vi "xcorr bkp nico SR.vi"(4 "shift":u8, 5 "Pulse Energy":fxp<+,32,0>=0.99609375, 6 "N":u8, 7 "y":u32, 8 "x":u32, 9 "enable":bool, 10 "lag":u16) -> (1 "Rxy valid":bool, 2 "Rxy":u64, 3 "trigger":bool)   [LabVIEW 2017]
uses:
  <vilib>/rvi/FXPMathLib/basic elements/FxpDiscreteDelay/XNode/nifxpmath_DiscreteDelay.xnode
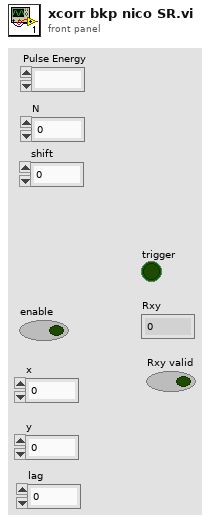
[diagram p1: front panel]
types:
  T1 = cluster{"Q[0]":bool, "Q[1]":bool, "Q[2]":bool, "Q[3]":bool, "Q[4]":bool, "Q[5]":bool, "Q[6]":bool, "Q[7]":bool, "Q[8]":bool, "Q[9]":bool, "Q[10]":bool, "Q[11]":bool, "Q[12]":bool}
  T2 = cluster{"out":u64, "Q":u64, "Q":u64, "Q":u64, "Q":u64, "Q":u64, "Q":u64, "Q":u64, "Q":u64, "Q":u64, "Q":u64, "Q":u64, "Q":u64}
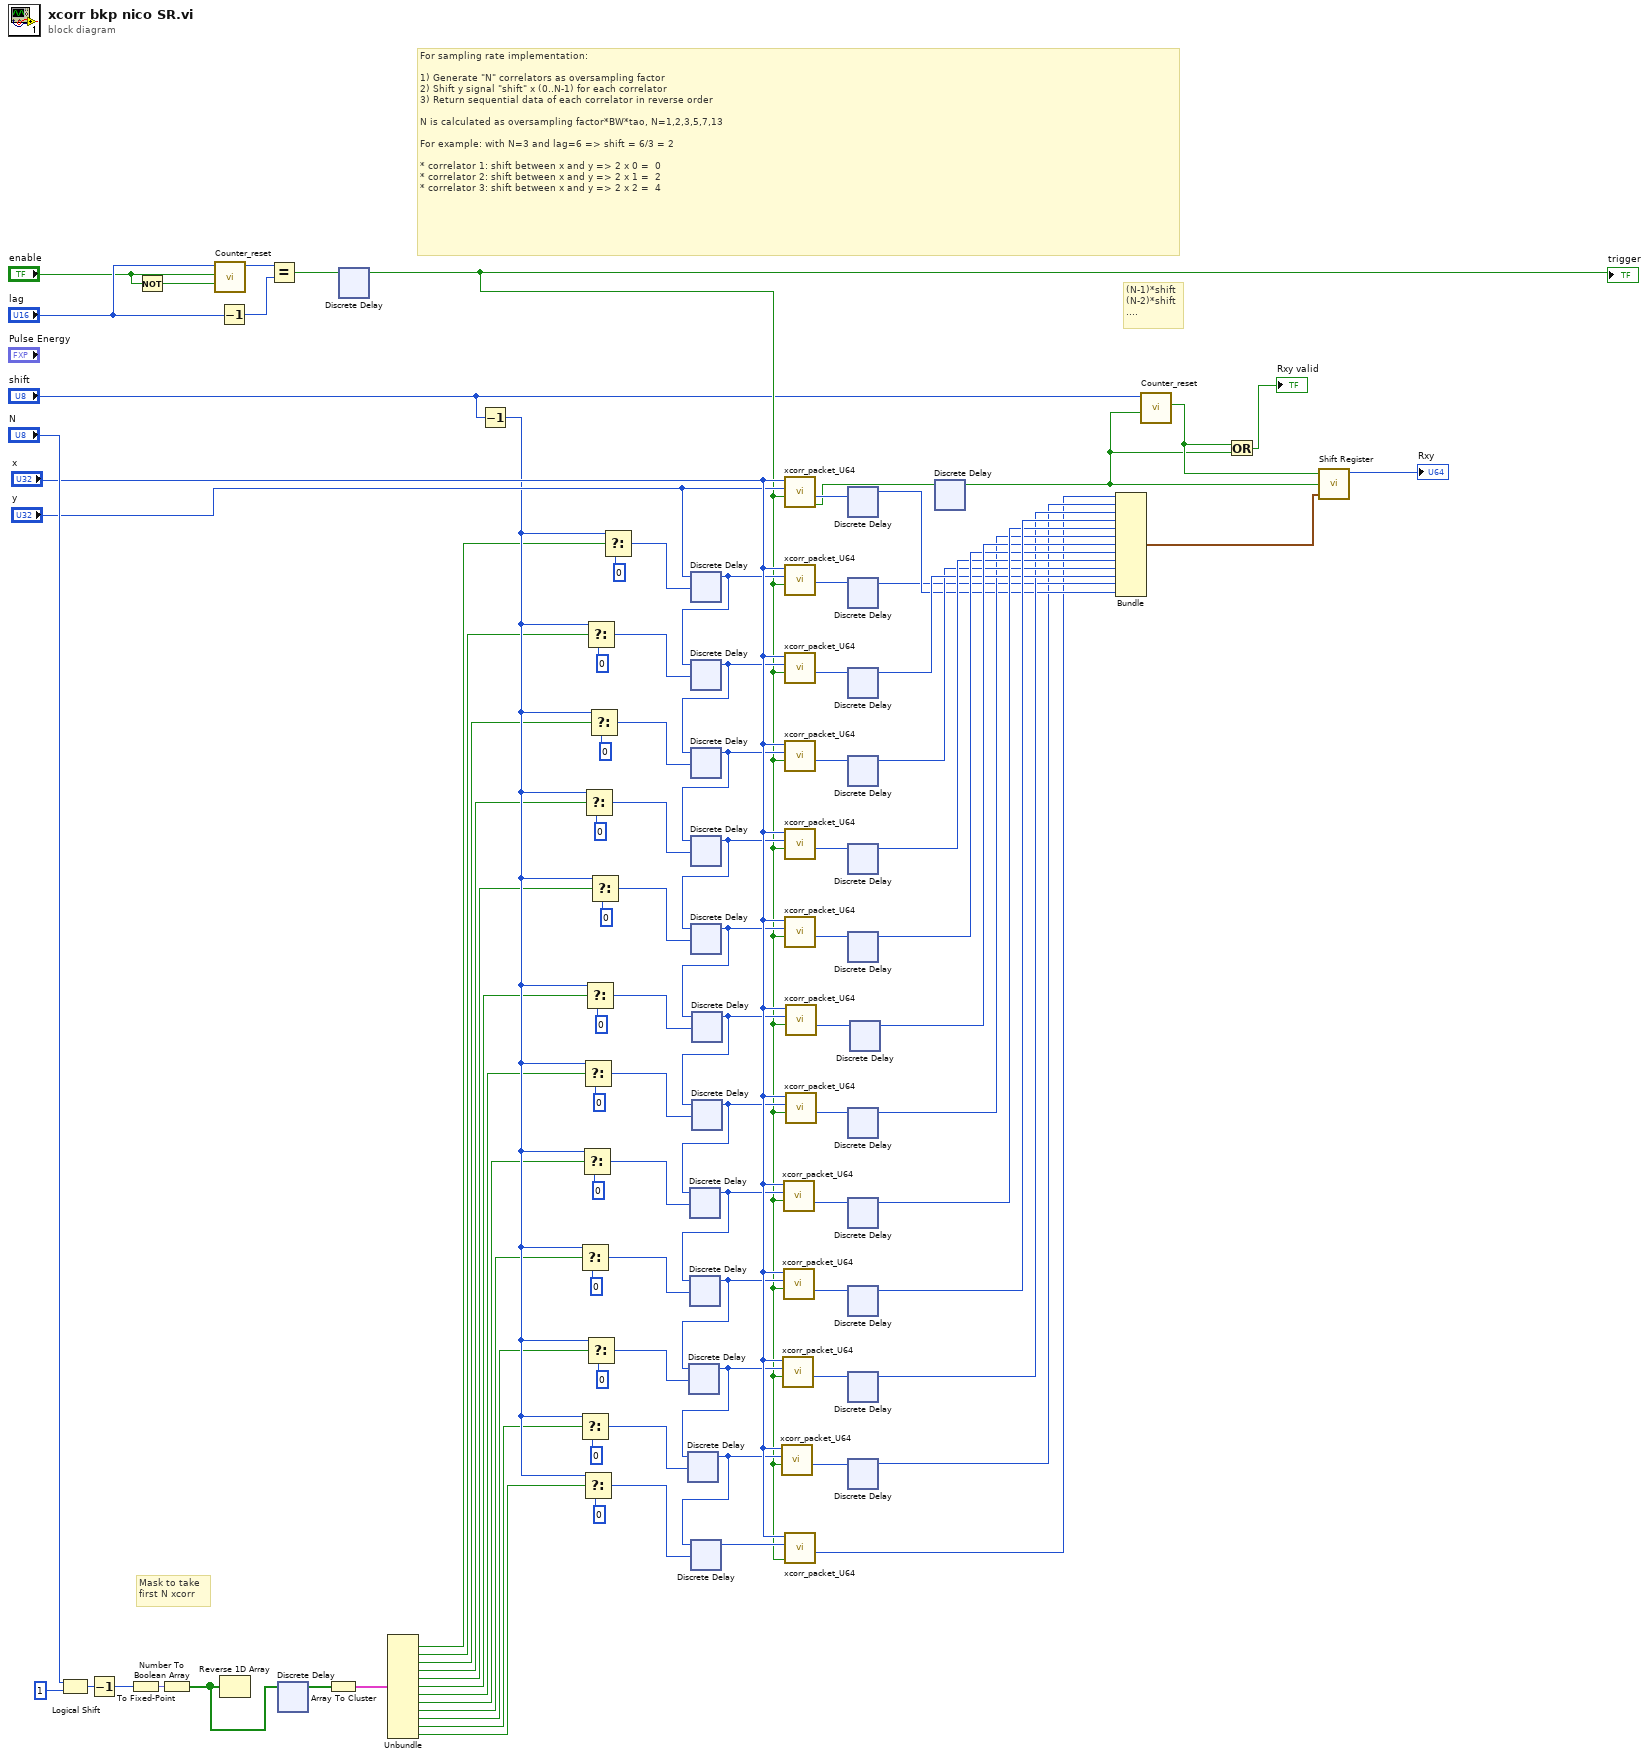
[diagram p0: block diagram]
diagram:
  # "(N-1)*shift\n(N-2)*shift\n...."
  # "Mask to take \nfirst N xcorr"
  # "For sampling rate implementation:\n\n1) Generate \"N\" correlators as oversampling factor\n2) Shift y signal \"shift\" x (0..N-1) for each correlator\n3) Return sequential data of each correlator in reverse order\n\nN is calculated as oversampling factor*BW*tao, N=1,2,3,5,7,13\n\nFor example: with N=3 and lag=6 => shift = 6/3 = 2\n\n* correlator 1: shift between x and y => 2 x 0 =  0\n* correlator 2: shift between x and y => 2 x 1 =  2\n* correlator 3: shift between x and y => 2 x 2 =  4"
  n1 = Logical Shift(y="N", x=u16 1) -> (x << y=w92:u16)
  n2 = Decrement(x=w92) -> (x-1=w91:u16)
  n3 = To Fixed-Point(number=w91) -> (fixed-point=w90:fxp<+,13,13>)  [unwired: 1 in]
  n4 = Not(x="enable") -> (.not. x?=w97:bool)
  n5 = Number To Boolean Array(number=w90) -> (Boolean array=w5:bool[])
  n6 = call "Counter_reset.vi"("reset"=w97, "enable"="enable", "limit"="lag") -> ("count"=w98:u16)  [unwired: 7 in, 1 out]
  n7 = Decrement(x="lag") -> (x-1=w96:u16)
  n8 = Reverse 1D Array(array=w5) -> ()  [unwired: 1 out]
  n9 = Equal?(x=w98, y=w96) -> (x = y?=w70:bool)
  n10 = xnode ("Discrete Delay")("D"=w5) -> ("Q"=w27:bool[])
  n11 = Array To Cluster(array=w27) -> (cluster=w69:T1)
  n12 = xnode ("Discrete Delay")("D"=w70) -> ("Q"=w61:bool)
  "trigger" <- w61
  n13 = Unbundle(w69) -> ("Q[1]"=w15:bool, "Q[2]"=w16:bool, "Q[3]"=w17:bool, "Q[4]"=w18:bool, "Q[5]"=w19:bool, "Q[6]"=w20:bool, "Q[7]"=w21:bool, "Q[8]"=w22:bool, "Q[9]"=w23:bool, "Q[10]"=w24:bool, "Q[11]"=w25:bool, "Q[12]"=w26:bool)  [unwired: 1 out]
  n14 = Decrement(x="shift") -> (x-1=w42:u8)
  n15 = Select(t=w42, s=w23, f=u8 0) -> (s? t:f=w47:u8)
  n16 = Select(t=w42, s=w25, f=u8 0) -> (s? t:f=w45:u8)
  n17 = Select(t=w42, s=w22, f=u8 0) -> (s? t:f=w48:u8)
  n18 = Select(t=w42, s=w21, f=u8 0) -> (s? t:f=w49:u8)
  n19 = Select(t=w42, s=w26, f=u8 0) -> (s? t:f=w44:u8)
  n20 = Select(t=w42, s=w18, f=u8 0) -> (s? t:f=w60:u8)
  n21 = Select(t=w42, s=w20, f=u8 0) -> (s? t:f=w50:u8)
  n22 = Select(t=w42, s=w16, f=u8 0) -> (s? t:f=w63:u8)
  n23 = Select(t=w42, s=w24, f=u8 0) -> (s? t:f=w46:u8)
  n24 = Select(t=w42, s=w17, f=u8 0) -> (s? t:f=w62:u8)
  n25 = Select(t=w42, s=w19, f=u8 0) -> (s? t:f=w51:u8)
  n26 = Select(t=w42, s=w15, f=u8 0) -> (s? t:f=w64:u8)
  n27 = xnode ("Discrete Delay")("D"="y", "n-1[0..255]"=w64) -> ("Q"=w75:u32)
  n28 = xnode ("Discrete Delay")("D"=w75, "n-1[0..255]"=w63) -> ("Q"=w85:u32)
  n29 = xnode ("Discrete Delay")("D"=w85, "n-1[0..255]"=w62) -> ("Q"=w84:u32)
  n30 = xnode ("Discrete Delay")("D"=w84, "n-1[0..255]"=w60) -> ("Q"=w83:u32)
  n31 = xnode ("Discrete Delay")("D"=w83, "n-1[0..255]"=w51) -> ("Q"=w82:u32)
  n32 = xnode ("Discrete Delay")("D"=w82, "n-1[0..255]"=w50) -> ("Q"=w81:u32)
  n33 = xnode ("Discrete Delay")("D"=w81, "n-1[0..255]"=w49) -> ("Q"=w80:u32)
  n34 = xnode ("Discrete Delay")("D"=w80, "n-1[0..255]"=w48) -> ("Q"=w79:u32)
  n35 = xnode ("Discrete Delay")("D"=w79, "n-1[0..255]"=w47) -> ("Q"=w78:u32)
  n36 = xnode ("Discrete Delay")("D"=w78, "n-1[0..255]"=w46) -> ("Q"=w77:u32)
  n37 = xnode ("Discrete Delay")("D"=w77, "n-1[0..255]"=w45) -> ("Q"=w76:u32)
  n38 = xnode ("Discrete Delay")("D"=w76, "n-1[0..255]"=w44) -> ("Q"=w86:u32)
  n39 = call "xcorr_packet_U64.vi"("x"="x", "y"=w76, "trigger"=w61) -> ("out"=w6:u64)  [unwired: 5 in, 1 out]
  n40 = call "xcorr_packet_U64.vi"("x"="x", "y"=w77, "trigger"=w61) -> ("out"=w8:u64)  [unwired: 5 in, 1 out]
  n41 = call "xcorr_packet_U64.vi"("x"="x", "y"=w79, "trigger"=w61) -> ("out"=w10:u64)  [unwired: 5 in, 1 out]
  n42 = call "xcorr_packet_U64.vi"("x"="x", "y"=w78, "trigger"=w61) -> ("out"=w9:u64)  [unwired: 5 in, 1 out]
  n43 = call "xcorr_packet_U64.vi"("x"="x", "y"="y", "trigger"=w61) -> ("out"=w31:u64, "valid"=w30:bool)  [unwired: 5 in]
  n44 = call "xcorr_packet_U64.vi"("x"="x", "y"=w75, "trigger"=w61) -> ("out"=w28:u64)  [unwired: 5 in, 1 out]
  n45 = call "xcorr_packet_U64.vi"("x"="x", "y"=w85, "trigger"=w61) -> ("out"=w32:u64)  [unwired: 5 in, 1 out]
  n46 = call "xcorr_packet_U64.vi"("x"="x", "y"=w84, "trigger"=w61) -> ("out"=w14:u64)  [unwired: 5 in, 1 out]
  n47 = call "xcorr_packet_U64.vi"("x"="x", "y"=w83, "trigger"=w61) -> ("out"=w34:u64)  [unwired: 5 in, 1 out]
  n48 = call "xcorr_packet_U64.vi"("x"="x", "y"=w82, "trigger"=w61) -> ("out"=w37:u64)  [unwired: 5 in, 1 out]
  n49 = call "xcorr_packet_U64.vi"("x"="x", "y"=w86, "trigger"=w61) -> ("out"=w1:u64)  [unwired: 5 in, 1 out]
  n50 = call "xcorr_packet_U64.vi"("x"="x", "y"=w81, "trigger"=w61) -> ("out"=w39:u64)  [unwired: 5 in, 1 out]
  n51 = call "xcorr_packet_U64.vi"("x"="x", "y"=w80, "trigger"=w61) -> ("out"=w12:u64)  [unwired: 5 in, 1 out]
  n52 = xnode ("Discrete Delay")("D"=w31) -> ("Q"=w4:u64)
  n53 = xnode ("Discrete Delay")("D"=w28) -> ("Q"=w3:u64)
  n54 = xnode ("Discrete Delay")("D"=w32) -> ("Q"=w33:u64)
  n55 = xnode ("Discrete Delay")("D"=w14) -> ("Q"=w13:u64)
  n56 = xnode ("Discrete Delay")("D"=w34) -> ("Q"=w35:u64)
  n57 = xnode ("Discrete Delay")("D"=w37) -> ("Q"=w36:u64)
  n58 = xnode ("Discrete Delay")("D"=w12) -> ("Q"=w11:u64)
  n59 = xnode ("Discrete Delay")("D"=w10) -> ("Q"=w40:u64)
  n60 = xnode ("Discrete Delay")("D"=w9) -> ("Q"=w41:u64)
  n61 = xnode ("Discrete Delay")("D"=w8) -> ("Q"=w7:u64)
  n62 = xnode ("Discrete Delay")("D"=w6) -> ("Q"=w2:u64)
  n63 = xnode ("Discrete Delay")("D"=w39) -> ("Q"=w38:u64)
  n64 = xnode ("Discrete Delay")("D"=w30) -> ("Q"=w29:bool)
  n65 = Bundle("out"=w1, "Q"=w2, "Q"=w7, "Q"=w41, "Q"=w40, "Q"=w11, "Q"=w38, "Q"=w36, "Q"=w35, "Q"=w13, "Q"=w33, "Q"=w3, "Q"=w4) -> (w74:T2)  [unwired: 1 in]
  n66 = call "Counter_reset.vi"("reset"=w29, "limit"="shift") -> ("count = limit?"=w71:bool)  [unwired: 8 in, 1 out]
  n67 = Or(x=w71, y=w29) -> (x .or. y?=→"Rxy valid":bool)
  n68 = call "Shift Register.vi"("Rxy in"=w74, "load"=w29, "shift"=w71) -> ("Rxy out"=→"Rxy":u64)  [unwired: 5 in]
